vi "Set DC Current Ramp to Zero.vi"(0 "Address":string="24", 1 "Current":dbl format="%.3e") -> ()   [LabVIEW 2012]
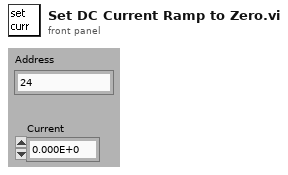
[diagram p1: front panel]
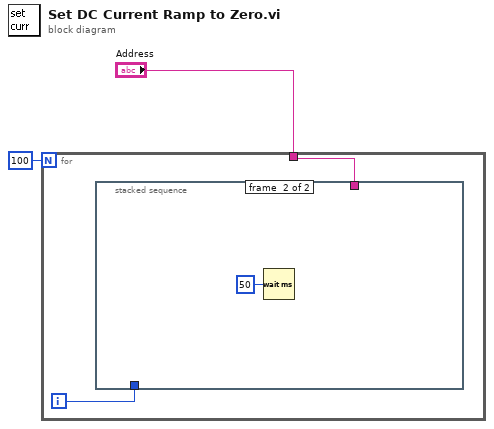
[diagram p0: block diagram]
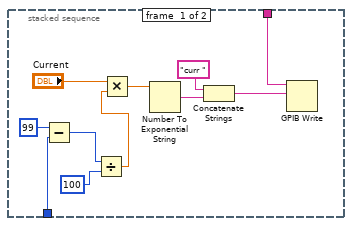
[diagram p2: hidden frame]
diagram:
  n1 = for {
    N: 100 -> [_]
    tunnel: "Address" -> [w4]
    i -> [w3]
    n2 = stacked-sequence {
      tunnel: w4 -> [w12 _]
      tunnel: w3 -> [w7 _]
      frame #0 {
        n3 = Subtract(x=99, y=w7) -> (x-y=w5:i32)
        n4 = Divide(x=w5, y=100) -> (x/y=w10:dbl)
        n5 = Multiply(x="Current", y=w10) -> (x*y=w9:dbl)
        n6 = Number To Exponential String(number=w9) -> (E-format string=w14:string)  [unwired: 3 in]
        n7 = Concatenate Strings("curr " ("string"), w14) -> (w13:string)
        n8 = GPIB Write(0:w12, 1:w13) -> ()  [unwired: 3 in, 2 out]
      }
      frame #1 {
        n9 = Wait (ms)(milliseconds to wait=u32 50) -> ()  [unwired: 1 out]
      }
    }
  }
